vi "Calculate Delta Angle.vi"(8 "Degrees 0-1":dbl=26.0, 10 "Distance (ft)":dbl(slide) scale=0.0..30.0, 11 "X":dbl(slide) scale=-1.0..1.0) -> (3 "Output Angle Delta":dbl=10.814159292035399)   [LabVIEW 2011]
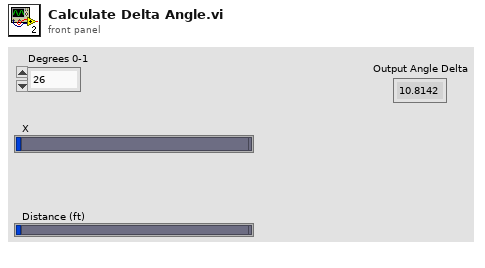
[diagram p1: front panel]
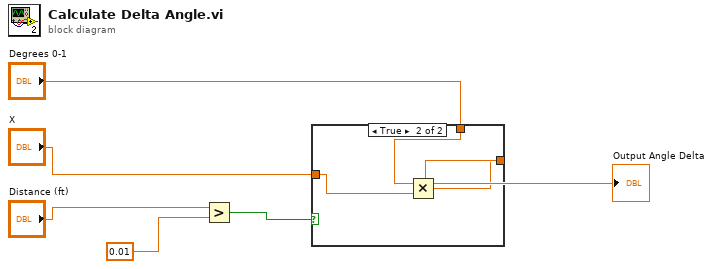
[diagram p0: block diagram]
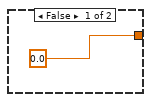
[diagram p2: hidden frame]
diagram:
  n1 = Greater?(x="Distance (ft)", y=0.01) -> (0:w4:bool)
  n2 = case shown="True" w4 {
    tunnel: [0.0 w8] -> w3
    tunnel: "X" -> [_ w10]
    tunnel: "Degrees 0-1" -> [_ w9]
    frame False {
    }
    frame True {
      n3 = Multiply(x=w9, y=w10) -> (x*y=w8:dbl)
    }
  }
  "Output Angle Delta" <- w3
